vi "Half Speed Drive.vi"(8 "R In":dbl, 9 "Y In":dbl, 10 "X In":dbl, 11 "Half Speed":bool) -> (1 "R Out":dbl, 2 "Y Out":dbl, 3 "X Out":dbl)   [LabVIEW 2014]
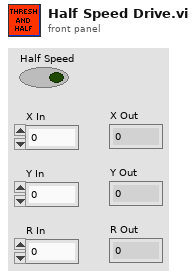
[diagram p1: front panel]
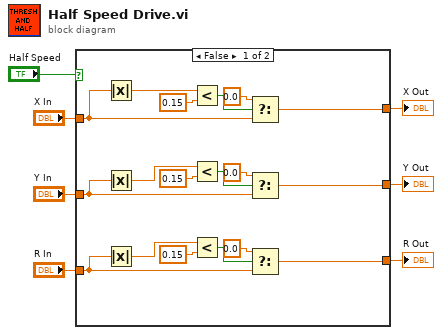
[diagram p0: block diagram]
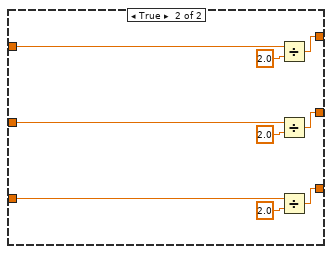
[diagram p2: hidden frame]
diagram:
  n1 = case shown="False" "Half Speed" {
    tunnel: [w20 w28] -> w5
    tunnel: "X In" -> [w21 w29]
    tunnel: "Y In" -> [w15 w30]
    tunnel: [w14 w27] -> w6
    tunnel: "R In" -> [w9 w31]
    tunnel: [w8 w26] -> w7
    frame False {
      n2 = Absolute Value(x=w21) -> (abs(x)=w25:dbl)
      n3 = Absolute Value(x=w15) -> (abs(x)=w19:dbl)
      n4 = Absolute Value(x=w9) -> (abs(x)=w10:dbl)
      n5 = Less?(x=w25, y=0.15) -> (x < y?=w23:bool)
      n6 = Less?(x=w19, y=0.15) -> (x < y?=w17:bool)
      n7 = Less?(x=w10, y=0.15) -> (x < y?=w12:bool)
      n8 = Select(t=0.0, s=w23, f=w21) -> (s? t:f=w20:dbl)
      n9 = Select(t=0.0, s=w17, f=w15) -> (s? t:f=w14:dbl)
      n10 = Select(t=0.0, s=w12, f=w9) -> (s? t:f=w8:dbl)
    }
    frame True {
      n11 = Divide(x=w29, y=2.0) -> (x/y=w28:dbl)
      n12 = Divide(x=w30, y=2.0) -> (x/y=w27:dbl)
      n13 = Divide(x=w31, y=2.0) -> (x/y=w26:dbl)
    }
  }
  "X Out" <- w5
  "Y Out" <- w6
  "R Out" <- w7
